vi "distance.vi"() -> ()   [LabVIEW 2015]
panel:
  out "A*B":dbl
  out "Tank":dbl(slide) scale=0.0..10.0
  out "Gauge":dbl(knob) scale=0.0..10.0
  in  "Slide":i16(slide) scale=0.0..10.0
  out "current time":timestamp
  out "String":string
  in  "stop":bool
  in  "Combo Box":string(combo)
  out "两点间距离":dbl
  in  "第二个点Y":dbl
  in  "第二个点X":dbl
  in  "第一个点Y":dbl
  in  "第一个点X":dbl
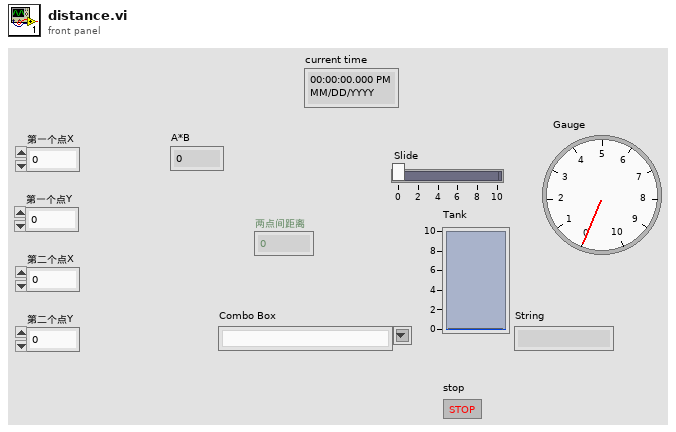
[diagram p1: front panel]
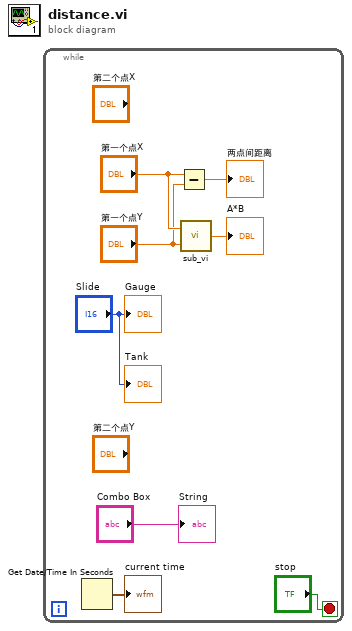
[diagram p0: block diagram]
diagram:
  n1 = while {
    stop <- "stop" stop-if-true
    n2 = Get Date/Time In Seconds() -> (seconds since 1Jan1904=→"current time":timestamp)
    n3 = Subtract(x="第一个点X", y="第一个点Y") -> (x-y=→"两点间距离":dbl)
    n4 = call "sub_vi.vi"("B"="第一个点Y", "A"="第一个点X") -> ("C"=→"A*B":dbl)
    "String" <- "Combo Box"
    "Gauge" <- "Slide"
    "Tank" <- "Slide"
  }
